vi "Get SD Normal Mode Channels.vi"(8 "error in (no error)":errorcluster, 11 "SD Module in":refnum<class "SD Module.lvclass">) -> (0 "error out":errorcluster, 1 "Channels":T2, 2 "Channel Names":string[](array[string]), 3 "SD Module out":refnum<class "SD Module.lvclass">, 4 "Type":T1)   [LabVIEW 2019, in "Modules.lvlib" / "SD Module.lvclass"]
uses:
  SD Module.lvclass
  RSI Module/Channels.ctl
  RSI Module/Channel Type.ctl
  <vilib>/NI VeriStand/Custom Device API/Custom Device Channel Type.ctl
  SD Module.lvclass/SD Module.ctl
  RSI Module/RSI Module.lvclass
  <vilib>/NI VeriStand/Custom Device API/Custom Device API.lvlib
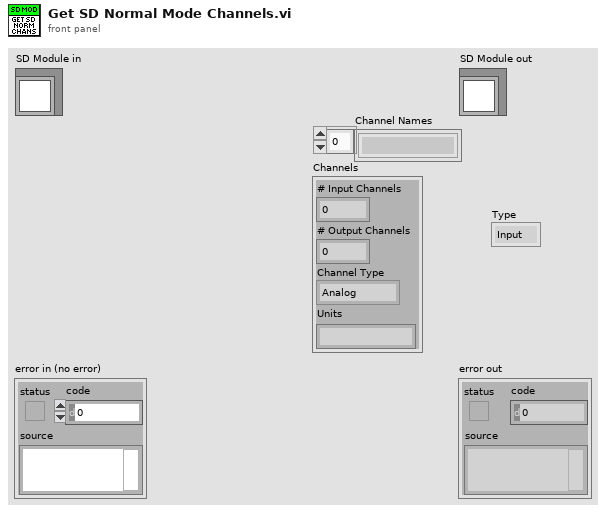
[diagram p1: front panel]
types:
  T1 = typedef "Custom Device API.lvlib/Custom Device Channel Type.ctl" = enum16{"Input", "Output"}
  T2 = typedef "Modules.lvlib/RSI Module.lvclass/Channels.ctl" = cluster{"# Input Channels":i32, "# Output Channels":i32, "Channel Type":T3, "Units":string}
  T3 = typedef "Modules.lvlib/RSI Module.lvclass/Channel Type.ctl" = enum16{"Analog", "Digital"}
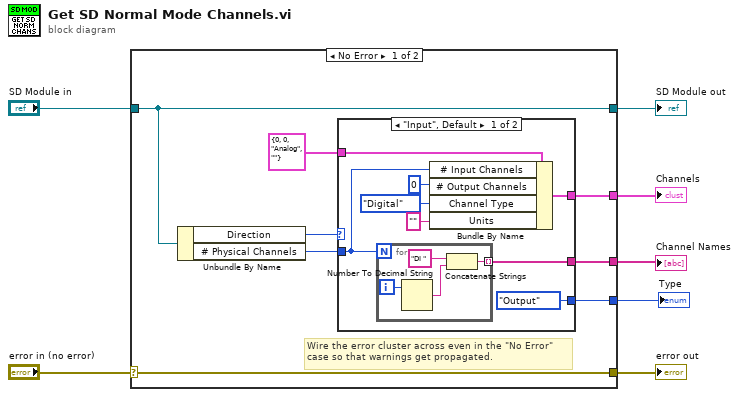
[diagram p0: block diagram]
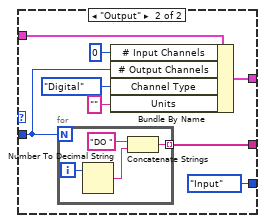
[diagram p2: hidden frame]
diagram:
  n1 = case shown="No Error" "error in (no error)" {
    selector: "error in (no error)" -> [w15 w41]
    tunnel: [w15 w41] -> w6
    tunnel: [w14 w40] -> w4
    tunnel: "SD Module in" -> [w14 w40]
    tunnel: [w10 _] -> w3
    tunnel: [w9 _] -> w2
    tunnel: [w8 _] -> w1
    frame No Error {
      # "Wire the error cluster across even in the \"No Error\"\ncase so that warnings get propagated."
      n2 = Unbundle By Name(w14) -> ("Direction"=w13:enum16{"Input", "Output", "Input/Output"}, "# Physical Channels"=w12:i32)
      n3 = case shown="\"Input\", Default" w13 {
        tunnel: w12 -> [w19 w31]
        tunnel: T2 {"# Input Channels"=0, "# Output Channels"=0, "Channel Type"=enum."Analog", "Units"=""} ("Channels") -> [w21 w33]
        tunnel: [w18 w32] -> w10
        tunnel: [w17 w29] -> w9
        tunnel: [Custom_Device_Channel_Type."Output" ("Type") Custom_Device_Channel_Type."Input" ("Type")] -> w8
        frame "Input", Default {
          n4 = for {
            N: w19 -> [_]
            tunnel: [w24] -> w17 mode=indexing
            i -> [w27]
            n5 = Number To Decimal String(number=w27) -> (decimal integer string=w25:string)  [unwired: 1 in]
            n6 = Concatenate Strings("DI ", w25) -> (w24:string)
          }
          n7 = Bundle By Name(cluster=w21, "# Input Channels"=w19, "# Output Channels"=0, "Channel Type"=Channel_Type."Digital", "Units"="") -> (w18:T2)
        }
        frame "Output" {
          n8 = for {
            N: w31 -> [_]
            tunnel: [w36] -> w29 mode=indexing
            i -> [w39]
            n9 = Number To Decimal String(number=w39) -> (decimal integer string=w37:string)  [unwired: 1 in]
            n10 = Concatenate Strings("DO ", w37) -> (w36:string)
          }
          n11 = Bundle By Name(cluster=w33, "# Input Channels"=0, "# Output Channels"=w31, "Channel Type"=Channel_Type."Digital", "Units"="") -> (w32:T2)
        }
      }
    }
    frame Error {
    }
  }
  "error out" <- w6
  "SD Module out" <- w4
  "Channel Names" <- w2
  "Channels" <- w3
  "Type" <- w1
